vi "Dll wrapper.vi"(7 "match_lengths (T)":bool=TRUE, 8 "error in (no error)":errorcluster, 10 "X":dbl[](array[numeric]), 11 "Y":dbl[](array[numeric])) -> (0 "error out":errorcluster, 1 "intercept":dbl, 2 "slope":dbl, 3 "Y_out":dbl[](array[numeric]), 4 "error":i32)   [LabVIEW 2021]
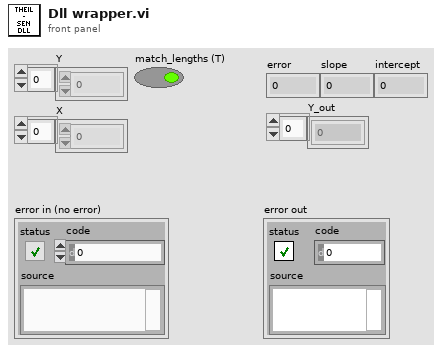
[diagram p1: front panel]
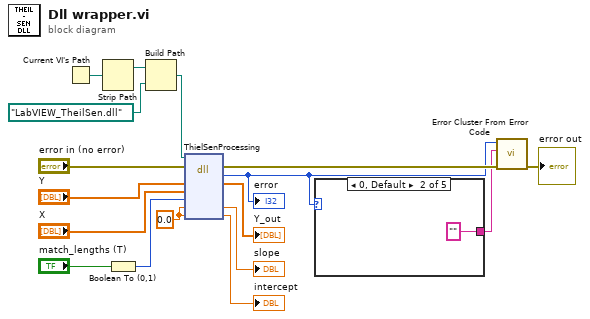
[diagram p0: block diagram]
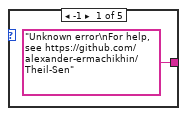
[diagram p2: hidden frame]
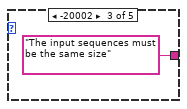
[diagram p3: hidden frame]
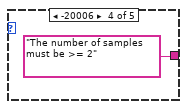
[diagram p4: hidden frame]
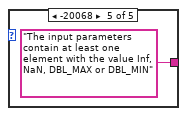
[diagram p5: hidden frame]
diagram:
  w13 = 0.0 ("slope")
  n1 = Current VI's Path() -> (path=w2:path)
  n2 = Strip Path(path=w2) -> (stripped path=w1:path)  [unwired: 1 out]
  n3 = Boolean To (0,1)(Boolean="match_lengths (T)") -> (0, 1=w15:i16)
  n4 = Build Path(base path=w1, name or relative path=path "LabVIEW_TheilSen.dll") -> (appended path=w3:path)
  n5 = dll-call lib="LabVIEW_TheilSen.dll" fn="ThielSenProcessing"(path in=w3, error in="error in (no error)", "Y"="Y", "X"="X", "match_lengths"=w15, "slope"=w13, "intercept"=w13) -> (error out=w8:errorcluster, "error"=w6:i32, "Y"=→"Y_out":dbl[], "slope"=→"slope":dbl, "intercept"=→"intercept":dbl)  [unwired: 3 in, 1 out]
  "error" <- w6
  n6 = case shown="0, Default" w6 {
    tunnel: ["Unknown error\nFor help, see https://github.com/alexander-ermachikhin/Theil-Sen" "" "The input sequences must be the same size" "The number of samples must be >= 2" "The input parameters contain at least one element with the value Inf, NaN, DBL_MAX or DBL_MIN"] -> w5
    frame -1 {
    }
    frame 0, Default {
    }
    frame -20002 {
    }
    frame -20006 {
    }
    frame -20068 {
    }
  }
  n7 = call <vilib>:"Error Cluster From Error Code.vi"("error in (no error)"=w8, "error message (\"\")"=w5, "error code (0)"=w6) -> ("error out"=→"error out":errorcluster)  [unwired: 6 in]
